vi "Read iRFData.vi"(8 "error in (no error)":errorcluster, 11 "APDClass in":refnum<class "APDClass.lvclass">) -> (0 "error out":errorcluster, 2 "iRFData":T1, 3 "APDClass out":refnum<class "APDClass.lvclass">)   [LabVIEW 2020, in "APDClass.lvclass"]
uses:
  APDClass.lvclass
  iRFData.ctl
  APDClass.lvclass/APDClass.ctl
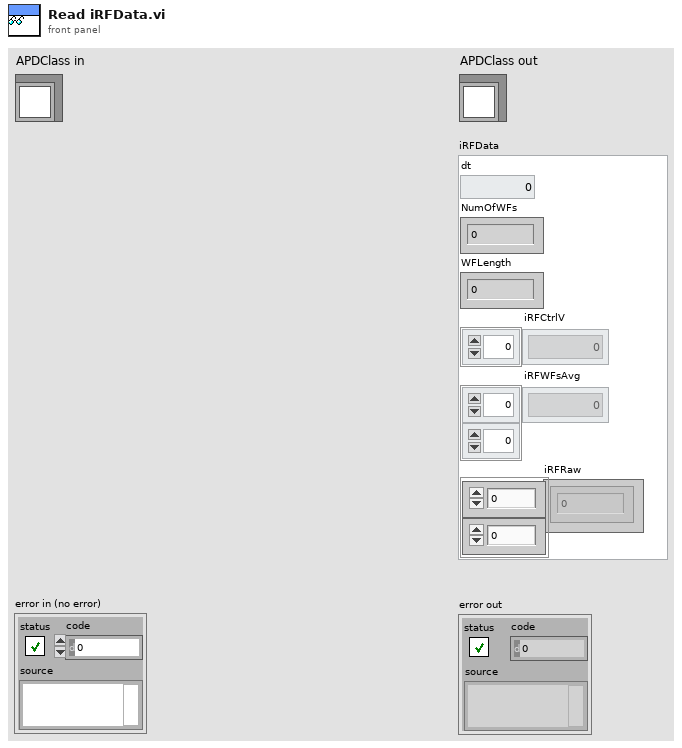
[diagram p1: front panel]
types:
  T1 = typedef "iRFData.ctl" = cluster{"dt":dbl, "NumOfWFs":i32, "WFLength":i32, "iRFCtrlV":dbl[], "iRFWFsAvg":dbl[][], "iRFRaw":dbl[][]}
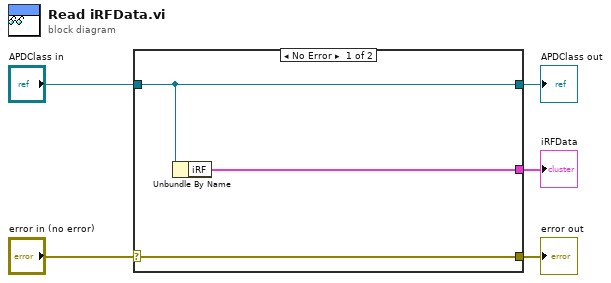
[diagram p0: block diagram]
diagram:
  n1 = case shown="No Error" "error in (no error)" {
    selector: "error in (no error)" -> [w8 w9]
    tunnel: [w8 w9] -> w4
    tunnel: [w7 w10] -> w2
    tunnel: "APDClass in" -> [w7 w10]
    tunnel: [w6 _] -> w1
    frame No Error {
      n2 = Unbundle By Name(w7) -> ("iRF"=w6:T1)
    }
    frame Error {
    }
  }
  "error out" <- w4
  "APDClass out" <- w2
  "iRFData" <- w1
